vi "Global _Stab_Profile.vi"() -> ()   [LabVIEW 2017]
panel:
  in  "Boolean":bool
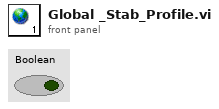
[diagram p1: front panel]
diagram:
